vi "Unpad Analyzer Region.vi"(4 "Analyzer Region":T2) -> (1 "Analyzer Region out":T1)   [LabVIEW 2018]
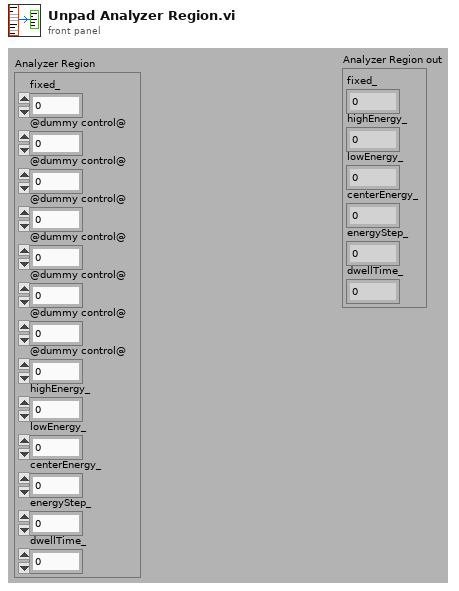
[diagram p1: front panel]
types:
  T1 = cluster{"fixed_":u8, "highEnergy_":dbl, "lowEnergy_":dbl, "centerEnergy_":dbl, "energyStep_":dbl, "dwellTime_":i32}
  T2 = cluster{"fixed_":u8, "@dummy control@":i8, "@dummy control@":i8, "@dummy control@":i8, "@dummy control@":i8, "@dummy control@":i8, "@dummy control@":i8, "@dummy control@":i8, "highEnergy_":dbl, "lowEnergy_":dbl, "centerEnergy_":dbl, "energyStep_":dbl, "dwellTime_":i32}
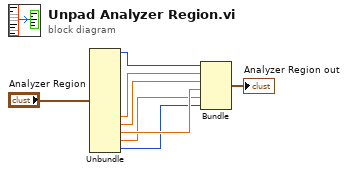
[diagram p0: block diagram]
diagram:
  n1 = Unbundle("Analyzer Region") -> ("fixed_"=w7:u8, "highEnergy_"=w6:dbl, "lowEnergy_"=w5:dbl, "centerEnergy_"=w4:dbl, "energyStep_"=w3:dbl, "dwellTime_"=w2:i32)  [unwired: 7 out]
  n2 = Bundle("fixed_"=w7, "highEnergy_"=w6, "lowEnergy_"=w5, "centerEnergy_"=w4, "energyStep_"=w3, "dwellTime_"=w2) -> (→"Analyzer Region out":T1)  [unwired: 1 in]
